vi "Calculate Target Data.vi"(8 "Rect Left":dbl, 9 "Rect Right":dbl, 10 "Distance to Target (ft)":dbl, 11 "Image Width (px)":dbl) -> (2 "X Location":dbl, 3 "Angle":dbl)   [LabVIEW 2012]
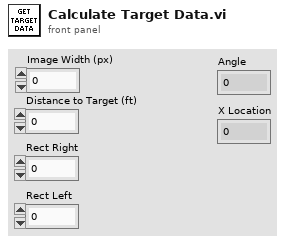
[diagram p1: front panel]
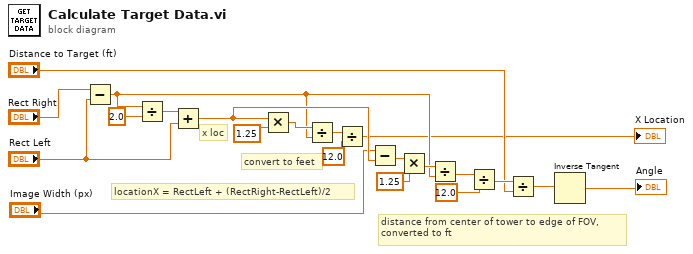
[diagram p0: block diagram]
diagram:
  # "distance from center of tower to edge of FOV, \nconverted to ft"
  # "x loc"
  # "convert to feet"
  # "locationX = RectLeft + (RectRight-RectLeft)/2"
  n1 = Subtract(x="Rect Right", y="Rect Left") -> (x-y=w11:dbl)
  n2 = Divide(x=w11, y=2.0) -> (x/y=w20:dbl)
  n3 = Add(x=w20, y="Rect Left") -> (x+y=w15:dbl)
  n4 = Multiply(x=w15, y=1.25) -> (x*y=w18:dbl)
  n5 = Divide(x=w18, y=w11) -> (x/y=w17:dbl)
  n6 = Divide(x=w17, y=12.0) -> (x/y=→"X Location":dbl)
  n7 = Subtract(x="Image Width (px)", y=w15) -> (x-y=w14:dbl)
  n8 = Multiply(x=w14, y=1.25) -> (x*y=w12:dbl)
  n9 = Divide(x=w12, y=w11) -> (x/y=w10:dbl)
  n10 = Divide(x=w10, y=12.0) -> (x/y=w8:dbl)
  n11 = Divide(x=w8, y="Distance to Target (ft)") -> (x/y=w7:dbl)
  n12 = Inverse Tangent(1:w7) -> (0:→"Angle":dbl)
